vi "Example Trigger Hold Mode.vi"() -> ()   [LabVIEW 2021]
doc: "This VI example shows how to use the Trigger hold mode of the instrument U1282A. It uses the Init, Abort and fetch blocks of the U1282A library to perform the trigger and reding of the measurement."
uses:
  Keysight U1282A.lvlib
panel:
  in  "VISA resource name":refnum<visa-resource-name>="Keysight_U1282A"
  in  "Salir":bool
  in  "Trigger":bool
  out "Reading":dbl
  # "This VI example allows the user to perform measurements using the Trigger Hold mode of the instrument U1282A. Use the Trigger button to execute a sequence of Trigger/Reading/Idle state. The reading of the primary display of the instrument is presented in the Reading indicator."
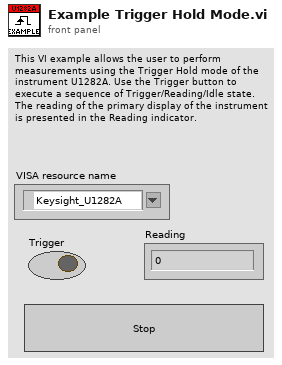
[diagram p1: front panel]
types:
  T1 = cluster{"Baud Rate":enum16{"1200", "2400", "4800", "9600", "19200", "38400", "57600", "115200"}, "Timeout":u32, "Stop Bits":u16, "Flow Control":enum16{"None", "XON / XOFF", "RTS / CTS", "DTR / DSR"}, "Parity":u16}
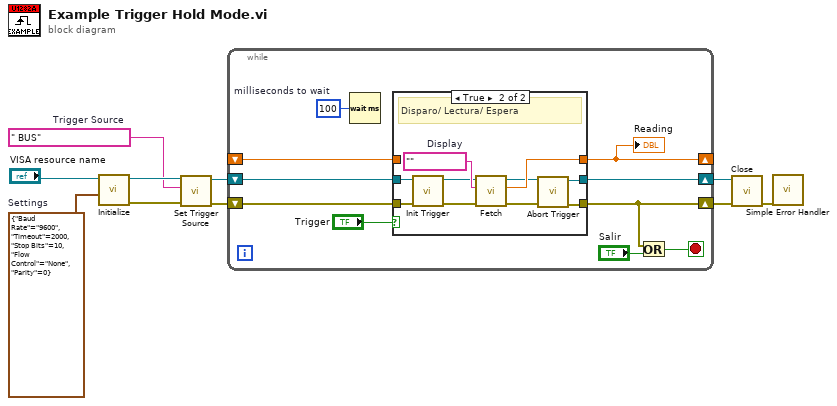
[diagram p0: block diagram]
diagram:
  w3 = T1 {"Baud Rate"=enum."9600", "Timeout"=2000, "Stop Bits"=10, "Flow Control"=enum."None", "Parity"=0}  # Settings
  w4 = " BUS"  # Trigger Source
  n1 = call "Initialize.vi"("Settings"=w3, "VISA resource name"="VISA resource name") -> ("error out"=w10:errorcluster, "VISA resource name out"=w9:refnum<visa-resource-name>)  [unwired: 8 in]
  n2 = call "Set Trigger Source.vi"("error in"=w10, "Trigger Source"=w4, "VISA resource name in"=w9) -> ("error out"=w6:errorcluster, "VISA resource name out"=w5:refnum<visa-resource-name>)  [unwired: 7 in]
  n3 = while {
    shift-right: [w14] -> w8
    shift-left: w6 -> [w18]
    shift-right: [w19] -> w7
    shift-left: w5 -> [w17]
    shift-right: [w15] -> _
    shift-left: _ -> [w16]
    stop <- w12 stop-if-true
    w11 = u32 100  # milliseconds to wait
    n4 = Wait (ms)(milliseconds to wait=w11) -> ()  [unwired: 1 out]
    n5 = case shown="True" "Trigger" {
      tunnel: [w22 w28] -> w14
      tunnel: [w23 w29] -> w19
      tunnel: w18 -> [w22 w33]
      tunnel: w17 -> [w23 w32]
      tunnel: w16 -> [w21 _]
      tunnel: [w21 w27] -> w15
      frame False {
      }
      frame True {
        w31 = ""  # Display
        # "Disparo/ Lectura/ Espera"
        n6 = call "Init Trigger.vi"("error in"=w33, "VISA resource name in"=w32) -> ("error out"=w24:errorcluster, "VISA resource name out"=w25:refnum<visa-resource-name>)  [unwired: 8 in]
        n7 = call "Fetch.vi"("error in"=w24, "Display"=w31, "VISA resource name in"=w25) -> ("error out"=w30:errorcluster, "Value"=w27:dbl, "VISA resource name out"=w26:refnum<visa-resource-name>)  [unwired: 6 in]
        n8 = call "Abort Trigger.vi"("error in"=w30, "VISA resource name in"=w26) -> ("error out"=w28:errorcluster, "VISA resource name out"=w29:refnum<visa-resource-name>)  [unwired: 8 in]
      }
    }
    "Reading" <- w15
    n9 = Or(x=w14, y="Salir") -> (x .or. y?=w12:bool)
  }
  n10 = call "Close.vi"("error in"=w8, "VISA resource name"=w7) -> ("error out"=w1:errorcluster)  [unwired: 9 in]
  n11 = call <vilib>:"Simple Error Handler.vi"("error in (no error)"=w1) -> ()  [unwired: 4 in, 5 out]
